vi "SetBSlope.vi"(0 "slope":u32=1, 1 "board_sel":u32=6) -> ()   [LabVIEW 2015]
uses:
  ESLSCDLL.dll
panel:
  # "1 for positive slope"
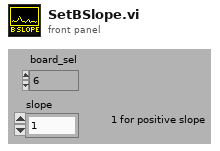
[diagram p1: front panel]
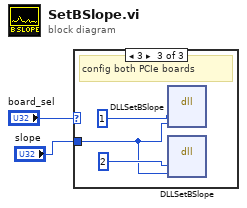
[diagram p0: block diagram]
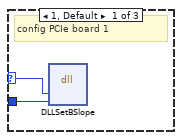
[diagram p2: hidden frame]
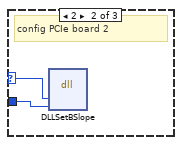
[diagram p3: hidden frame]
diagram:
  n1 = case shown="3" "board_sel" {
    selector: "board_sel" -> [w3 w6 _]
    tunnel: "slope" -> [w4 w5 w7]
    frame 1, Default {
      # "config PCIe board 1"
      n2 = dll-call lib="C:/Users/flori/Nextcloud/Dokumente/Stresing/Windows/lv64/board.vis/ESLSCDLL.dll" fn="DLLSetBSlope" ("lwlscdll.dll:DLLSetTemp")("drv"=w3, "slope"=w4) -> ()  [unwired: 6 in, 2 out]
    }
    frame 2 {
      # "config PCIe board 2"
      n3 = dll-call lib="C:/Users/flori/Nextcloud/Dokumente/Stresing/Windows/lv64/board.vis/ESLSCDLL.dll" fn="DLLSetBSlope" ("lwlscdll.dll:DLLSetTemp")("drv"=w6, "slope"=w5) -> ()  [unwired: 6 in, 2 out]
    }
    frame 3 {
      # "config both PCIe boards"
      n4 = dll-call lib="C:/Users/flori/Nextcloud/Dokumente/Stresing/Windows/lv64/board.vis/ESLSCDLL.dll" fn="DLLSetBSlope" ("lwlscdll.dll:DLLSetTemp")("drv"=u32 1, "slope"=w7) -> ()  [unwired: 6 in, 2 out]
      n5 = dll-call lib="C:/Users/flori/Nextcloud/Dokumente/Stresing/Windows/lv64/board.vis/ESLSCDLL.dll" fn="DLLSetBSlope" ("lwlscdll.dll:DLLSetTemp")("drv"=u32 2, "slope"=w7) -> ()  [unwired: 6 in, 2 out]
    }
  }
